vi "LVClass_WavefrontCorrectorSet Get Files Destination.vi"(0 "WavefrontCorrectorSet in":refnum<class "WavefrontCorrectorSet.lvclass">, 5 "repertoire":path, 11 "error in (no error)":errorcluster) -> (4 "WavefrontCorrectorSet out":refnum<class "WavefrontCorrectorSet.lvclass">, 15 "error out":errorcluster)   [LabVIEW 2020, in "WavefrontCorrectorSet.lvclass"]
uses:
  WavefrontCorrectorSet.lvclass
  WavefrontCorrectorSet.lvclass/WavefrontCorrectorSet.ctl
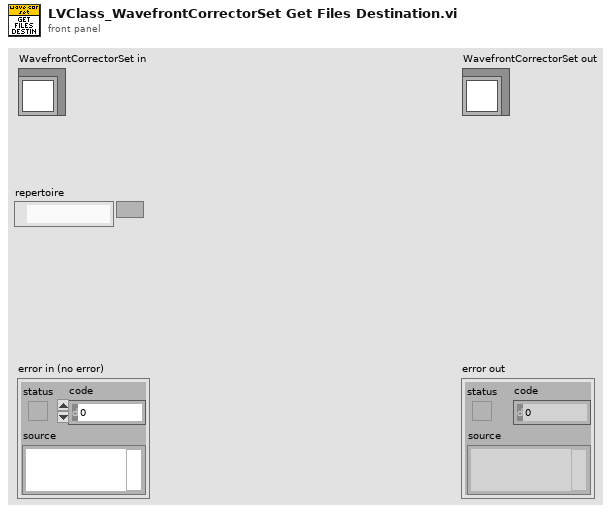
[diagram p1: front panel]
types:
  T1 = typedef "WavefrontCorrectorSpecifications.ctl" = cluster{"Mirror name":string, "Plugin name":string, "Serial number":string, "Revision":string, "Number of commands":i32, "Sleep after command apply (ms)":i32, "Has internal memory ?":bool}
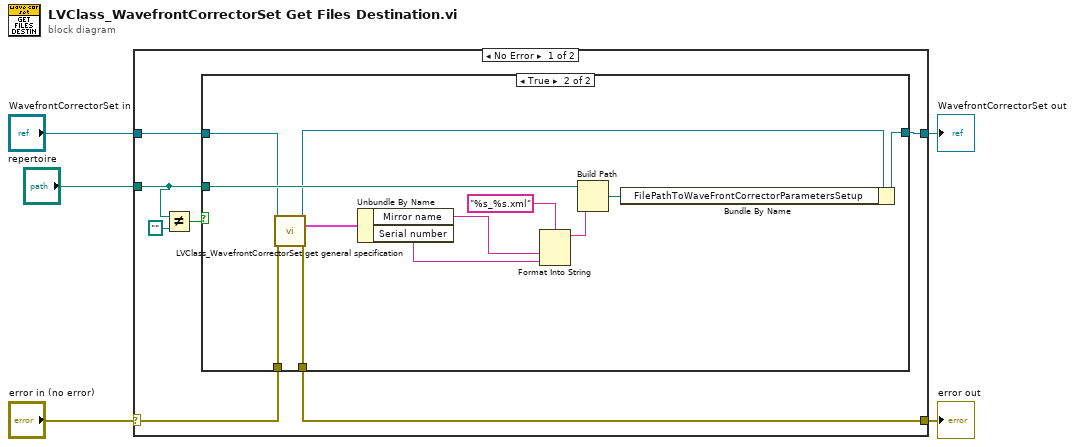
[diagram p0: block diagram]
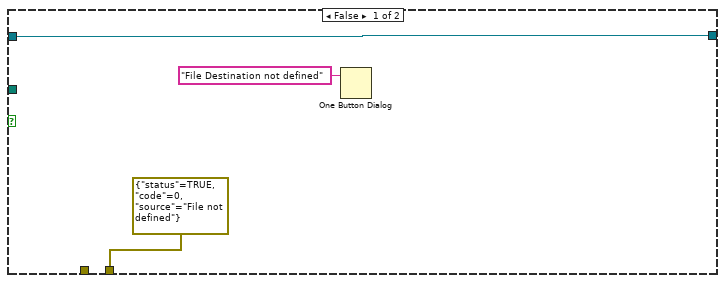
[diagram p2: hidden frame]
diagram:
  n1 = case shown="No Error" "error in (no error)" {
    selector: "error in (no error)" -> [w12 w29]
    tunnel: [w11 w29] -> w4
    tunnel: [w9 w28] -> w2
    tunnel: "WavefrontCorrectorSet in" -> [w10 w28]
    tunnel: "repertoire" -> [w6 _]
    frame No Error {
      n2 = Not Equal?(x=w6, y=path "") -> (x != y?=w7:bool)
      n3 = case shown="True" w7 {
        tunnel: w12 -> [_ w19]
        tunnel: [errorcluster {"status"=TRUE, "code"=0, "source"="File not defined"} ("error out") w18] -> w11
        tunnel: w10 -> [w13 w20]
        tunnel: w6 -> [_ w27]
        tunnel: [w13 w26] -> w9
        frame False {
          n4 = One Button Dialog(message="File Destination not defined") -> ()  [unwired: 1 in, 1 out]
        }
        frame True {
          n5 = call "LVClass_WavefrontCorrectorSet get general specification.vi"("WavefrontCorrectorSet in"=w20, "error in (no error)"=w19) -> ("WavefrontCorrectorSet out"=w17:refnum<class "WavefrontCorrectorSet.lvclass">, "ConfigMiroir"=w16:T1, "error out"=w18:errorcluster)  [unwired: 11 in]
          n6 = Unbundle By Name(w16) -> ("Mirror name"=w23:string, "Serial number"=w22:string)
          n7 = Format Into String(format string="%s_%s.xml", w23, w22) -> (resulting string=w21:string)  [unwired: 2 in, 1 out]
          n8 = Build Path(base path=w27, name or relative path=w21) -> (appended path=w25:path)
          n9 = Bundle By Name(cluster=w17, "FilePathToWaveFrontCorrectorParametersSetup"=w25) -> (w26:refnum<class "WavefrontCorrectorSet.lvclass">)
        }
      }
    }
    frame Error {
    }
  }
  "error out" <- w4
  "WavefrontCorrectorSet out" <- w2
